vi "Clear Fault Configuration.vi"(0 "target address (localhost)":string="localhost", 1 "code to clear":i32, 3 "error in (no error)":errorcluster) -> (10 "error out":errorcluster)   [LabVIEW 2020, in "Config Faults.lvlib"]
doc: "Clears the custom fault configuration for a configurable fault and applies the default configuration."
uses:
  <vilib>/NIScanEngine/ConfigurableFaults/Config Faults.lvlib
  <resource>/objmgr/ni.var.rc
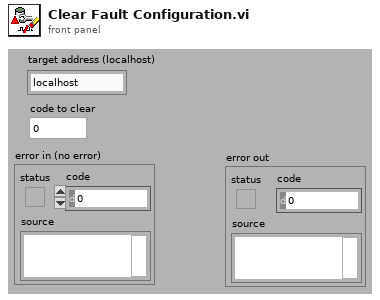
[diagram p1: front panel]
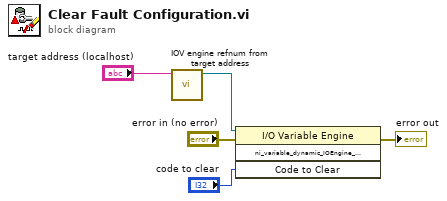
[diagram p0: block diagram]
diagram:
  n1 = call <vilib>:"IOV engine refnum from target address.vi"("target address"="target address (localhost)") -> ("reference out"=w4:refnum<k21>)  [unwired: 10 in]
  n2 = invoke class="I/O Variable Engine" method="ni_variable_dynamic_IOEngine_ClearFaultConfig"(reference=w4, error in="error in (no error)", "Code to Clear"="code to clear") -> (error out=→"error out":errorcluster)  [unwired: 1 in, 3 out]
